vi "CompileFrontPanel.vi"(8 "error in":errorcluster, 11 "RasPi Compiler in":refnum<class "RasPi Compiler.lvclass">) -> (0 "error out":errorcluster, 3 "RasPi Compiler out":refnum<class "RasPi Compiler.lvclass">)   [LabVIEW 2014, in "Raspberry Pi Compatible Compiler for LabVIEW.lvlib" / "RasPi Compiler.lvclass"]
uses:
  RasPi Compiler.lvclass
  RasPi Compiler.lvclass/RasPi Compiler.ctl
  Python/PythonConverter_GUI/PythonConverter_GUI.lvclass
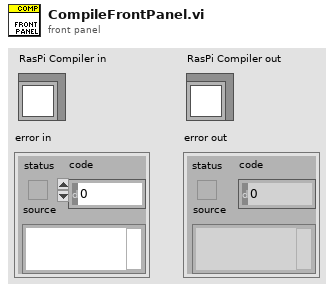
[diagram p1: front panel]
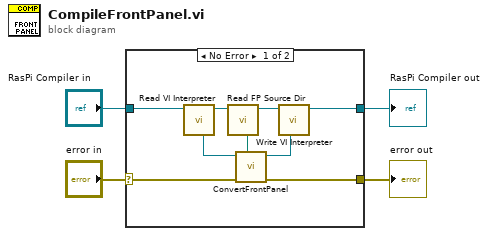
[diagram p0: block diagram]
diagram:
  n1 = case shown="No Error" "error in" {
    selector: "error in" -> [w9 w15]
    tunnel: [w8 w15] -> w3
    tunnel: [w6 w14] -> w1
    tunnel: "RasPi Compiler in" -> [w10 w14]
    frame No Error {
      n2 = call "Read VI Interpreter.vi"("RasPi Compiler in"=w10) -> ("RasPi Compiler out"=w11:refnum<class "RasPi Compiler.lvclass">, "VI Interpreter"=w12:refnum<class "VI Interpreter.lvclass">)  [unwired: 7 in]
      n3 = call "Read FP Source Dir.vi"("RasPi Compiler in"=w11) -> ("RasPi Compiler out"=w5:refnum<class "RasPi Compiler.lvclass">, "FP Source Dir"=w13:path)  [unwired: 7 in]
      n4 = call "ConvertFrontPanel.vi"("Build Directory"=w13, "error in"=w9, "VI Interpreter"=w12) -> ("error out"=w8:errorcluster, "VI Interpreter out"=w7:refnum<class "VI Interpreter.lvclass">)  [unwired: 7 in]
      n5 = call "Write VI Interpreter.vi"("VI Interpreter"=w7, "RasPi Compiler in"=w5) -> ("RasPi Compiler out"=w6:refnum<class "RasPi Compiler.lvclass">)  [unwired: 7 in]
    }
    frame Error {
    }
  }
  "error out" <- w3
  "RasPi Compiler out" <- w1
